vi "Teleop.vi"(10 "Match Info":T1={"Autonomous Elapsed Seconds"=0.0, "TeleOp Elapsed Seconds"=0.0, "Disabled Elapsed Seconds"=0.0, "Visited Autonomous"=FALSE, "Visited TeleOp"=FALSE, "Visited Disabled"=FALSE, "Autonomous Settings"={"Autonomous Style"=enum."Independent", "VI Refnum"=refnum}}, 11 "Call Context":T2) -> ()   [LabVIEW 2013]
doc: "This VI is called for each TeleOp packet received from the DS where the robot is not disabled. It is often used to read from the joysticks and update I/O or to update setpoints for timed control loops. It should complete and return within 20 milliseconds or it may miss DS packets."
uses:
  <vilib>/Rock Robotics/WPI/DriverStation/WPI_DriverStationDerivedRobotMode.ctl
  <vilib>/Rock Robotics/WPI/DriverStation/WPI_DriverStationMatch Info.ctl
  Robot Global Data.vi
  Systems/Drive/Drive Global.vi
  Systems/Intake/Intake Global.vi
  Systems/Cannon/Cannon Global.vi
  <vilib>/Rock Robotics/WPI/Joystick/WPI_JoystickGetSetRefNum.vi
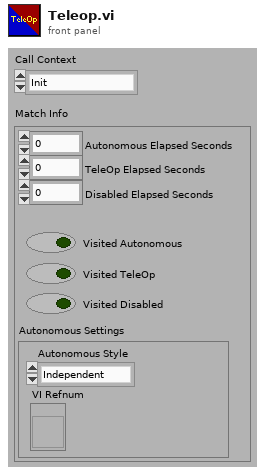
[diagram p1: front panel]
types:
  T1 = typedef "WPI_DriverStationMatch Info.ctl" = cluster{"Autonomous Elapsed Seconds":dbl, "TeleOp Elapsed Seconds":dbl, "Disabled Elapsed Seconds":dbl, "Visited Autonomous":bool, "Visited TeleOp":bool, "Visited Disabled":bool, "Autonomous Settings":cluster{"Autonomous Style":enum16{"Iterative", "Independent"}, "VI Refnum":refnum<vi>}}
  T2 = typedef "WPI_DriverStationDerivedRobotMode.ctl" = enum16{"Init", "Execute", "Stop"}
  T3 = typedef "WPI_JoystickDevRef.ctl" = cluster{"Device":T4}
  T4 = typedef "WPI_JoystickDeviceEnum.ctl" = enum16{"USB 1", "USB 2", "USB 3", "USB 4", "Kinect 1", "Kinect 2"}
  T5 = typedef "WPI_JoystickButtonState.ctl" = cluster{"Button 1":bool, "Button 2":bool, "Button 3":bool, "Button 4":bool, "Button 5":bool, "Button 6":bool, "Button 7":bool, "Button 8":bool, "Button 9":bool, "Button 10":bool, "Button 11":bool, "Button 12":bool}
  T6 = cluster{"axis 1 (x)":dbl, "axis 2 (y)":dbl, "axis 3 (throttle)":dbl, "axis 4":dbl, "axis 5":dbl, "axis 6":dbl}
  T7 = typedef "WPI_SolenoidValue.ctl" = enum16{"Off", "On", "Forward", "Reverse"}
  T8 = cluster{"Intake Execute":T7, "Gripper Execute":T7, "Gripper In":dbl, "Intake Arm":dbl}
  T9 = cluster{"V - Bus out":dbl, "Manual Power In":dbl, "Stop Auto?":bool, "Ball":bool, "Catch":bool, "Low Point":bool, "Catcher":T7, "Change Catcher?":bool}
  T10 = cluster{"X - Axis":dbl, "Y - Axis":dbl, "Slow Drive?":bool, "Right Side RPM":dbl, "Right Side Distance":dbl, "Left Side RPM ":dbl, "Left Side Distance":dbl}
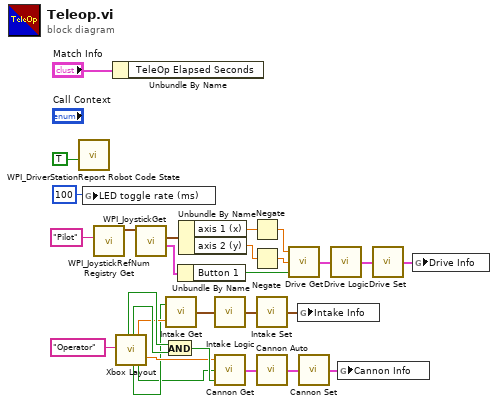
[diagram p0: block diagram]
diagram:
  n1 = call <vilib>:"WPI_DriverStationReport Robot Code State.vi"("TeleOp"=TRUE ("Autonomous")) -> ()  [unwired: 10 in, 1 out]
  n2 = global write "Robot Global Data.vi" "LED toggle rate (ms)"(u32 100 ("LED ms toggle rate")) -> ()
  n3 = call <vilib>:"WPI_JoystickRefNum Registry Get.vi"("refnum name"="Pilot") -> ("JoystickDevRef"=w23:T3)  [unwired: 9 in, 1 out]
  n4 = Unbundle By Name("Match Info") -> ()  [unwired: 1 out]
  n5 = call "Xbox Layout.vi"("Joystick Name"="Operator") -> ("Left Button"=w11:bool, "Right Button"=w10:bool, "X"=w5:bool, "L+R Throttles"=w6:dbl, "Y"=w4:bool, "Right Stick Y"=w9:dbl)  [unwired: 3 in, 10 out]
  n6 = call <vilib>:"WPI_JoystickGet.vi"("JoystickDevRef"=w23) -> ("Buttons"=w20:T5, "Axes"=w21:T6)  [unwired: 4 in, 1 out]
  n7 = And(x=w11, y=w10) -> (x .and. y?=w12:bool)
  n8 = call "Intake Get.vi"("Gripper"=w6, "Change arm?"=w5) -> ("Intake Info Out"=w3:T8)
  n9 = Unbundle By Name(w20) -> ("Button 1"=w19:bool)
  n10 = Unbundle By Name(w21) -> ("axis 1 (x)"=w17:dbl, "axis 2 (y)"=w18:dbl)
  n11 = call "Intake Logic.vi"("Intake Info In"=w3) -> ("Intake Info Out"=w8:T8)
  n12 = call "Cannon Get.vi"("Stop Auto?"=w12, "Change Catcher"=w4, "Cannon Power"=w9) -> ("Cannon Info Out"=w16:T9)
  n13 = Negate(x=w17) -> (-x=w2:dbl)
  n14 = Negate(x=w18) -> (-x=w1:dbl)
  n15 = call "Intake Set.vi"("Intake Info In"=w8) -> ("Intake Info Out"=w7:T8)
  n16 = call "Cannon Auto.vi"("Cannon Info In"=w16) -> ("Cannon Info Out"=w15:T9)
  n17 = call "Drive Get.vi"("Slow Drive?- In"=w19, "Axis - Y In"=w1, "Axis - X In"=w2) -> ("Drive Info Out"=w26:T10)
  n18 = global write "Intake Global.vi" "Intake Info"(w7) -> ()
  n19 = call "Cannon Set.vi"("Cannon Info In"=w15) -> ("Cannon Info Out"=w14:T9)
  n20 = call "Drive Logic.vi"("Drive Info  In"=w26) -> ("Drive Info Out"=w25:T10)
  n21 = global write "Cannon Global.vi" "Cannon Info"(w14) -> ()
  n22 = call "Drive Set.vi"("Drive Info In"=w25) -> ("Drive Info Out"=w24:T10)
  n23 = global write "Drive Global.vi" "Drive Info"(w24) -> ()
